vi "U8_3_byte_Array_to_voltage_current_Rev02.vi"(0 "Nmbr_of_datapoints":dbl=128.0, 1 "Array In":u8[](array[numeric]), 4 "CH1 multiplier":dbl, 5 "CH0 multiplier":dbl, 6 "CH1 Shift V":dbl, 11 "AC/DC":bool, 12 "CH0 Shift V":dbl) -> (7 "HEXVAL":string, 8 "CH1RMS":dbl, 9 "CH2RMS":dbl, 10 "CH1 DC Shift":dbl, 13 "CH2 DC Shift":dbl, 14 "Loop count":dbl, 15 "Voltage":dbl[](graph), 16 "CH1DC":dbl, 17 "Current":dbl[](graph), 18 "mV":dbl, 19 "CH2DC":dbl)   [LabVIEW 2012]
uses:
  <vilib>/measure/madcrms.llb/Basic Averaged DC-RMS for 1 Chan.vi
  <vilib>/Analysis/5stat.llb/RMS (DBL).vi
  <vilib>/measure/NI_MAPro.lvlib
  <vilib>/Analysis/NI_AALPro.lvlib
panel:
  out "number of samples":dbl
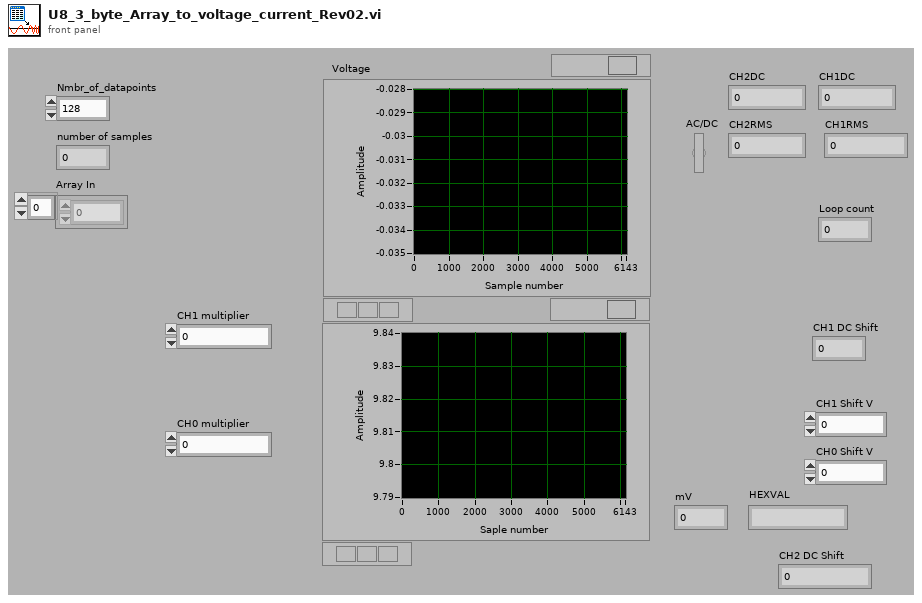
[diagram p1: front panel]
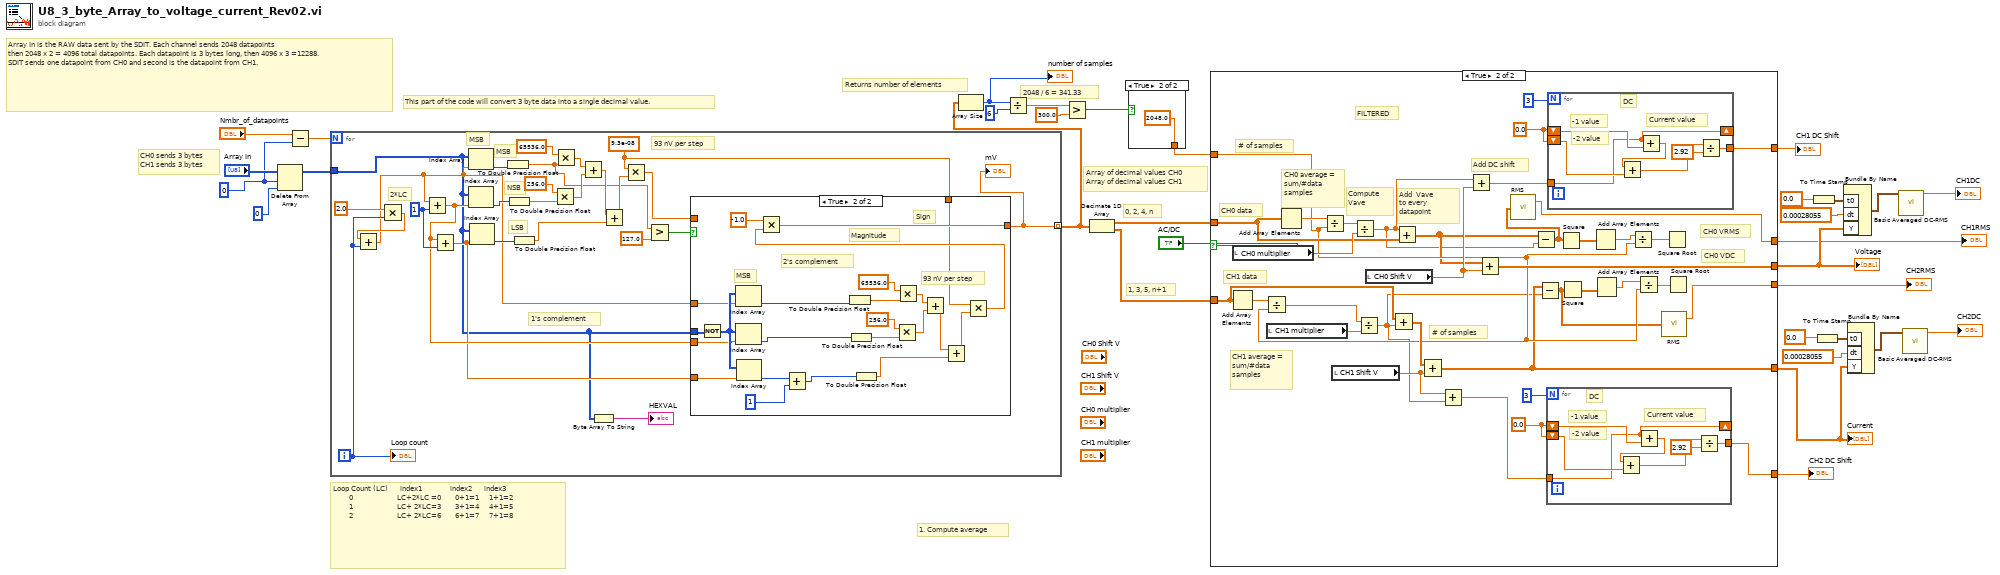
[diagram p0: block diagram]
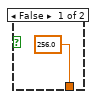
[diagram p2: hidden frame]
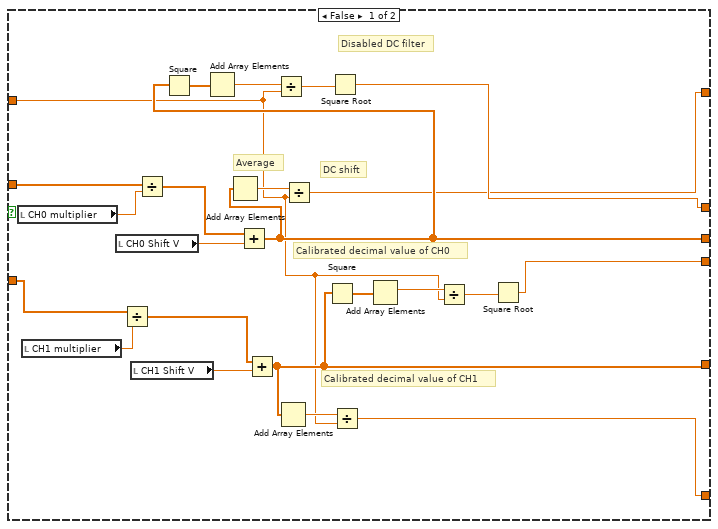
[diagram p3: hidden frame]
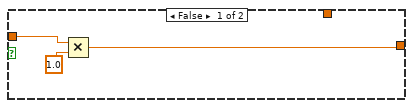
[diagram p4: hidden frame]
diagram:
  w28 = 0
  # "Array In is the RAW data sent by the SDIT. Each channel sends 2048 datapoints\nthen 2048 x 2 = 4096 total datapoints. Each datapoint is 3 bytes long, then 4096 x 3 =12288.\nSDIT sends one datapoint from CH0 and second is the datapoint from CH1."
  # "Returns number of elements"
  # "This part of the code will convert 3 byte data into a single decimal value."
  # "2048 / 6 = 341.33"
  # "1. Compute average"
  # "1, 3, 5, n+1"
  # "0, 2, 4, n"
  # "Array of decimal values CH0\nArray of decimal values CH1"
  # "CH0 sends 3 bytes\nCH1 sends 3 bytes"
  # "Loop Count (LC)      index1              index2      index3      \n        0                      LC+2*LC =0       0+1=1     1+1=2\n        1                      LC+ 2*LC=3       3+1=4     4+1=5\n        2                      LC+ 2*LC=6       6+1=7     7+1=8"
  n1 = Delete From Array(array="Array In", length=w28, index=0) -> (array with subset deleted=w27:u8[])  [unwired: 1 out]
  n2 = Subtract(x="Nmbr_of_datapoints", y=w28) -> (x-y=w30:dbl)
  n3 = for {
    N: w30 -> [_]
    tunnel: w27 -> [w34]
    tunnel: [w33] -> w18 mode=indexing
    i -> [w40]
    w39 = 9.3e-08
    w50 = 1
    # "93 nV per step"
    # "LSB"
    # "MSB"
    # "NSB"
    # "1's complement"
    # "MSB"
    # "2*LC"
    n4 = Multiply(x=2.0, y=w40) -> (x*y=w48:dbl)
    n5 = Add(x=w48, y=w40) -> (x+y=w38:dbl)
    n6 = Add(x=w38, y=w50) -> (x+y=w37:dbl)
    n7 = Add(x=w37, y=w50) -> (x+y=w36:dbl)
    n8 = Index Array(array=w34, index=w38) -> (element=w43:u8)
    n9 = Index Array(array=w34, index=w37) -> (element=w42:u8)
    n10 = Index Array(array=w34, index=w36) -> (element=w41:u8)
    n11 = To Double Precision Float(number=w43) -> (double precision float=w44:dbl)
    n12 = To Double Precision Float(number=w42) -> (double precision float=w56:dbl)
    n13 = To Double Precision Float(number=w41) -> (double precision float=w52:dbl)
    n14 = Multiply(x=256.0, y=w56) -> (x*y=w54:dbl)
    n15 = Multiply(x=65536.0, y=w44) -> (x*y=w58:dbl)
    n16 = Add(x=w58, y=w54) -> (x+y=w53:dbl)
    n17 = Byte Array To String(unsigned byte array=w34) -> (string=→"HEXVAL":string)
    n18 = Add(x=w53, y=w52) -> (x+y=w51:dbl)
    n19 = Multiply(x=w39, y=w51) -> (x*y=w47:dbl)
    n20 = Greater?(x=w44, y=127.0) -> (0:w46:bool)
    n21 = case shown="True" w46 {
      tunnel: [w61 w84] -> w33
      tunnel: w47 -> [w60 _]
      tunnel: w34 -> [_ w71]
      tunnel: w38 -> [_ w66]
      tunnel: w37 -> [_ w65]
      tunnel: w36 -> [_ w64]
      tunnel: w39 -> [_ w62]
      frame False {
        n22 = Multiply(x=w60, y=1.0) -> (x*y=w61:dbl)
      }
      frame True {
        # "93 nV per step"
        # "Magnitude"
        # "Sign"
        # "2's complement"
        # "MSB"
        n23 = Not(x=w71) -> (.not. x?=w70:u8[])
        n24 = Index Array(array=w70, index=w66) -> (element=w73:u8)
        n25 = Index Array(array=w70, index=w65) -> (element=w72:u8)
        n26 = Index Array(array=w70, index=w64) -> (element=w69:u8)
        n27 = Add(x=w69, y=1) -> (x+y=w67:i32)
        n28 = To Double Precision Float(number=w73) -> (double precision float=w74:dbl)
        n29 = To Double Precision Float(number=w72) -> (double precision float=w80:dbl)
        n30 = To Double Precision Float(number=w67) -> (double precision float=w76:dbl)
        n31 = Multiply(x=256.0, y=w80) -> (x*y=w78:dbl)
        n32 = Multiply(x=65536.0, y=w74) -> (x*y=w82:dbl)
        n33 = Add(x=w82, y=w78) -> (x+y=w77:dbl)
        n34 = Add(x=w77, y=w76) -> (x+y=w75:dbl)
        n35 = Multiply(x=w62, y=w75) -> (x*y=w63:dbl)
        n36 = Multiply(x=-1.0, y=w63) -> (x*y=w84:dbl)
      }
    }
    "mV" <- w33
    "Loop count" <- w40
  }
  n37 = Array Size(array=w18) -> (size(s)=w22:i32)
  "number of samples" <- w22
  n38 = Divide(x=w22, y=6) -> (x/y=w21:dbl)
  n39 = Greater?(x=w21, y=300.0) -> (0:w19:bool)
  n40 = Decimate 1D Array(w18) -> (w1:dbl[], w25:dbl[])
  n41 = case shown="True" w19 {
    tunnel: [256.0 2048.0] -> w17
    frame False {
    }
    frame True {
    }
  }
  n42 = case shown="True" "AC/DC" {
    tunnel: w1 -> [w101 w128]
    tunnel: w25 -> [w109 w127]
    tunnel: [w92 w116] -> w2
    tunnel: [w93 w124] -> w15
    tunnel: [w88 w131] -> w24
    tunnel: [w89 w136] -> w23
    tunnel: w17 -> [w90 w119]
    tunnel: [w100 w110] -> w4
    tunnel: [w94 w112] -> w3
    frame False {
      # "Disabled DC filter"
      # "Calibrated decimal value of CH1"
      # "Calibrated decimal value of CH0"
      # "DC shift"
      # "Average"
      n43 = local read "CH0 multiplier"() -> (w104:dbl)
      n44 = local read "CH1 multiplier"() -> (w108:dbl)
      n45 = local read "CH0 Shift V"() -> (w103:dbl)
      n46 = Divide(x=w109, y=w108) -> (x/y=w95:dbl[])
      n47 = local read "CH1 Shift V"() -> (w107:dbl)
      n48 = Divide(x=w101, y=w104) -> (x/y=w106:dbl[])
      n49 = Add(x=w106, y=w103) -> (x+y=w93:dbl[])
      n50 = Square(x=w93) -> (x^2=w102:dbl[])
      n51 = Add Array Elements(numeric array=w102) -> (sum=w87:dbl)
      n52 = Add Array Elements(numeric array=w93) -> (sum=w105:dbl)
      n53 = Add(x=w95, y=w107) -> (x+y=w92:dbl[])
      n54 = Divide(x=w87, y=w90) -> (x/y=w99:dbl)
      n55 = Add Array Elements(numeric array=w92) -> (sum=w91:dbl)
      n56 = Divide(x=w105, y=w90) -> (x/y=w89:dbl)
      n57 = Square(x=w92) -> (x^2=w98:dbl[])
      n58 = Square Root(x=w99) -> (sqrt(x)=w100:dbl)
      n59 = Divide(x=w91, y=w90) -> (x/y=w88:dbl)
      n60 = Add Array Elements(numeric array=w98) -> (sum=w96:dbl)
      n61 = Divide(x=w96, y=w90) -> (x/y=w97:dbl)
      n62 = Square Root(x=w97) -> (sqrt(x)=w94:dbl)
    }
    frame True {
      w133 = 0.0
      w138 = 0.0
      # "FILTERED"
      # "CH1 average = sum/#data samples"
      # "CH0 VRMS"
      # "CH0 VDC"
      # "Add DC shift"
      # "Compute Vave"
      # "# of samples"
      # "# of samples"
      # "CH1 data"
      # "CH0 data"
      # "Add  Vave\nto every datapoint"
      # "CH0 average = sum/#data samples"
      n63 = Add Array Elements(numeric array=w127) -> (sum=w143:dbl)
      n64 = local read "CH0 multiplier"() -> (w140:dbl)
      n65 = Divide(x=w143, y=w119) -> (x/y=w142:dbl)
      n66 = local read "CH1 multiplier"() -> (w139:dbl)
      n67 = Add Array Elements(numeric array=w128) -> (sum=w144:dbl)
      n68 = Divide(x=w144, y=w119) -> (x/y=w117:dbl)
      n69 = local read "CH1 Shift V"() -> (w130:dbl)
      n70 = Divide(x=w117, y=w140) -> (x/y=w114:dbl)
      n71 = Divide(x=w142, y=w139) -> (x/y=w115:dbl)
      n72 = local read "CH0 Shift V"() -> (w135:dbl)
      n73 = Add(x=w127, y=w115) -> (x+y=w141:dbl[])
      n74 = Add(x=w114, y=w128) -> (x+y=w118:dbl[])
      n75 = Add(x=w141, y=w130) -> (x+y=w116:dbl[])
      n76 = Add(x=w130, y=w115) -> (x+y=w129:dbl)
      n77 = Add(x=w114, y=w135) -> (x+y=w134:dbl)
      n78 = Add(x=w118, y=w135) -> (x+y=w124:dbl[])
      n79 = Subtract(x=w118, y=w114) -> (x-y=w111:dbl[])
      n80 = call-poly <vilib>:"RMS.vi"("X"=w111) -> ("rms value"=w110:dbl)  [unwired: 1 out]
      n81 = Subtract(x=w116, y=w115) -> (x-y=w113:dbl[])
      n82 = for {
        N: 3 -> [_]
        shift-right: [w145] -> _
        shift-left: w133 -> [w151]
        shift-left: w133 -> [w148]
        tunnel: [w146] -> w131
        tunnel: w129 -> [w145]
        # "DC"
        # "-2 value"
        # "-1 value"
        # "Current value"
        n83 = Add(x=w145, y=w151) -> (x+y=w149:dbl)
        n84 = Add(x=w149, y=w148) -> (x+y=w147:dbl)
        n85 = Divide(x=w147, y=2.92) -> (x/y=w146:dbl)
      }
      n86 = for {
        N: 3 -> [_]
        shift-right: [w152] -> _
        shift-left: w138 -> [w158]
        shift-left: w138 -> [w155]
        tunnel: [w153] -> w136
        tunnel: w134 -> [w152]
        # "DC"
        # "-2 value"
        # "-1 value"
        # "Current value"
        n87 = Add(x=w152, y=w158) -> (x+y=w156:dbl)
        n88 = Add(x=w156, y=w155) -> (x+y=w154:dbl)
        n89 = Divide(x=w154, y=2.92) -> (x/y=w153:dbl)
      }
      n90 = Square(x=w111) -> (x^2=w123:dbl[])
      n91 = Square(x=w113) -> (x^2=w120:dbl[])
      n92 = Add Array Elements(numeric array=w123) -> (sum=w125:dbl)
      n93 = Add Array Elements(numeric array=w120) -> (sum=w121:dbl)
      n94 = Divide(x=w125, y=w119) -> (x/y=w126:dbl)
      n95 = Divide(x=w121, y=w119) -> (x/y=w122:dbl)
      n96 = call-poly <vilib>:"RMS.vi"("X"=w113) -> ("rms value"=w112:dbl)  [unwired: 1 out]
      n97 = Square Root(x=w126) -> ()  [unwired: 1 out]
      n98 = Square Root(x=w122) -> ()  [unwired: 1 out]
    }
  }
  "Current" <- w2
  "Voltage" <- w15
  "CH2 DC Shift" <- w24
  "CH1 DC Shift" <- w23
  "CH1RMS" <- w4
  "CH2RMS" <- w3
  n99 = To Time Stamp(1:0.0 ("t0")) -> (0:w13:timestamp)
  n100 = To Time Stamp(1:0.0 ("t0")) -> (0:w9:timestamp)
  n101 = Bundle By Name("t0"=w13, "dt"=0.00028055, "Y"=w15) -> (w14:waveform(dbl))  [unwired: 1 in]
  n102 = Bundle By Name("t0"=w9, "dt"=0.00028055, "Y"=w2) -> (w10:waveform(dbl))  [unwired: 1 in]
  n103 = call-poly <vilib>:"Basic Averaged DC-RMS.vi"("signal in"=w14) -> ("DC value"=→"CH1DC":dbl)  [unwired: 7 in, 3 out]
  n104 = call-poly <vilib>:"Basic Averaged DC-RMS.vi"("signal in"=w10) -> ("DC value"=→"CH2DC":dbl)  [unwired: 7 in, 3 out]
